vi "Read.vi"(8 "error in (no error)":errorcluster, 11 "HAL in":refnum<class "HAL.lvclass">) -> (0 "error out":errorcluster, 2 "response":string, 3 "HAL out":refnum<class "HAL.lvclass">)   [LabVIEW 2019, in "HAL.lvclass"]
doc: "Override to <b>close</b> the connection to your hardware"
uses:
  HAL.lvclass
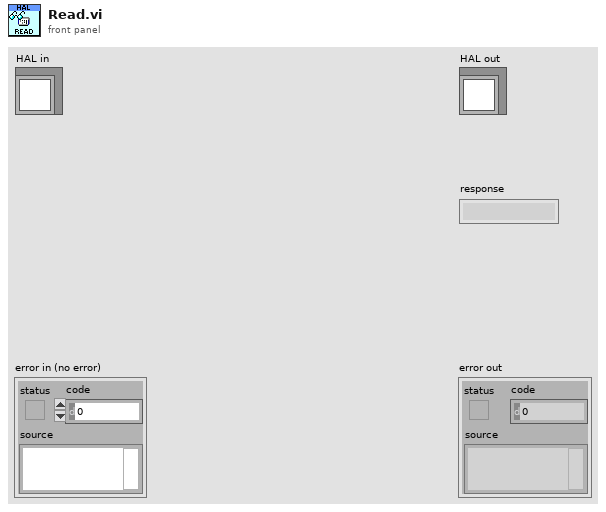
[diagram p1: front panel]
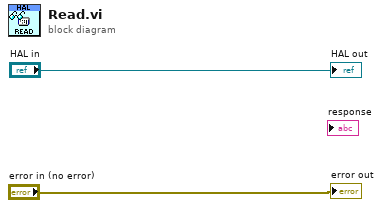
[diagram p0: block diagram]
diagram:
  "error out" <- "error in (no error)"
  "HAL out" <- "HAL in"
